vi "UEvent_SET_INTERNAL_EXTERNAL_POWER_SOURCE.vi"(6 "Ex/Int PW":T1(ring), 9 "USB":tag, 10 "Value":T2, 11 "Refnum in":refnum<k21>) -> (1 "Battery_Voltage":dbl, 2 "DUT_Voltage":dbl, 3 "Refnum out":refnum<k21>)   [LabVIEW 2015]
uses:
  Range_Shunt_selector.ctl
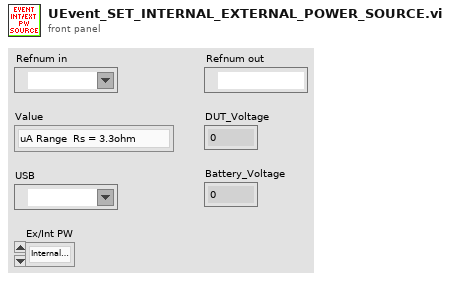
[diagram p1: front panel]
types:
  T1 = enum16{"Internal PW Source", "External PW Source"}
  T2 = typedef "Range_Shunt_selector.ctl" = enum16{"uA Range  Rs = 3.3ohm", "mA Range Rs = 3.3Ohm", "mA Range Rs = 1Ohm", "mA Range Rs = 1Ohm - X2"}
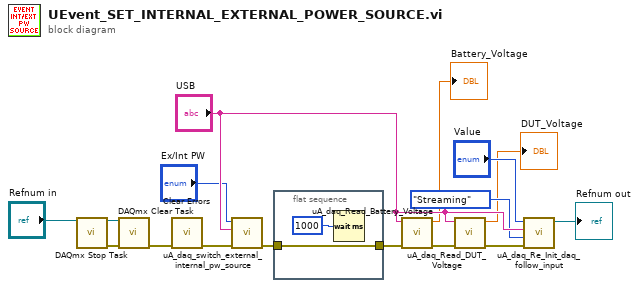
[diagram p0: block diagram]
diagram:
  n1 = call <vilib>:"DAQmx Stop Task.vi"("task/channels in"="Refnum in") -> ("task out"=w4:refnum<k21>, "error out"=w1:errorcluster)  [unwired: 13 in]
  n2 = call <vilib>:"DAQmx Clear Task.vi"("task in"=w4, "error in"=w1) -> ("error out"=w2:errorcluster)  [unwired: 13 in]
  n3 = call <vilib>:"Clear Errors.vi"("error in (no error)"=w2) -> ("error out"=w9:errorcluster)  [unwired: 5 in, 1 out]
  n4 = call "uA_daq_switch_external_internal_pw_source.vi"("error in"=w9, "USB DAQ"="USB", "Ex/Int PW"="Ex/Int PW") -> ("error out"=w10:errorcluster)  [unwired: 8 in]
  n5 = flat-sequence {
    tunnel: w10 -> [w17]
    tunnel: [w17] -> w11
    frame #0 {
      n6 = Wait (ms)(milliseconds to wait=u32 1000) -> ()  [unwired: 1 out]
    }
  }
  n7 = call "uA_daq_Read_Battery_Voltage.vi"("error in"=w11, "USB DAQ"="USB") -> ("error out"=w7:errorcluster, "Battery_Voltage"=→"Battery_Voltage":dbl)  [unwired: 8 in]
  n8 = call "uA_daq_Read_DUT_Voltage.vi"("error in"=w7, "USB DAQ"="USB") -> ("error out"=w16:errorcluster, "DUT_Voltage"=→"DUT_Voltage":dbl)  [unwired: 8 in]
  n9 = call "uA_daq_Re_Init_daq_follow_input.vi"("error in (no error)"=w16, "Acquire Mode"=enum16{"Streaming", "Read All", "Stop"}."Streaming", "USB"="USB", "Range_shunt"="Value") -> ("Refnum out"=→"Refnum out":refnum<k21>)  [unwired: 6 in, 1 out]
